vi "VariableValuesToClusters.vi"(11 "VariableValues":refnum<class "VariableValue.lvclass">[](array[class])) -> (3 "VariableValueClusters":cluster{"Name":string, "Value":dbl}[](array[cluster]))   [LabVIEW 2013, in "VariableManagerAPI.lvlib"]
uses:
  VariableManagerAPI.lvlib
  VariableValue/VariableValue.lvclass
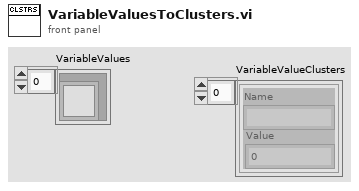
[diagram p1: front panel]
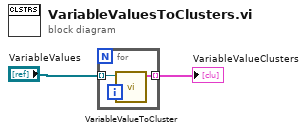
[diagram p0: block diagram]
diagram:
  n1 = for {
    tunnel: "VariableValues" -> [w4] mode=indexing
    tunnel: [w3] -> w1 mode=indexing
    n2 = call "VariableValueToCluster.vi"("VariableValue"=w4) -> ("VariableValueCluster"=w3:cluster{"Name":string, "Value":dbl})  [unwired: 10 in]
  }
  "VariableValueClusters" <- w1
